vi "MVC OOP Advanced with Commands.vi"() -> ()   [LabVIEW 2011]
doc: "This VI is a basic function generator utilising a class to encapsulate the frequency, type and resulatnt waveform. It also utilises the command pattern design pattern to control the program flow."
uses:
  Controls/Waveform Type.ctl
  Advanced Waveform Class/Advanced Waveform.lvclass
  Message Class/Message.lvclass
  Message Class/Stop Message/Stop Message.lvclass
  Message Class/Set Frequency Message/Set Frequency Message.lvclass
  Message Class/Waveform Type Message/Waveform Type Message.lvclass
  Message Class/Generate Signal Message/Generate Signal Message.lvclass
  Message Class/FFT Signal Message/FFT Signal Message.lvclass
panel:
  in  "Waveform Type":T1
  in  "FFT Signal":bool
  in  "Gen Signal":bool
  in  "Frequency":dbl(knob) scale=0.0..11.0
  out "Waveform Graph":waveform(dbl)(graph)
  in  "stop":bool
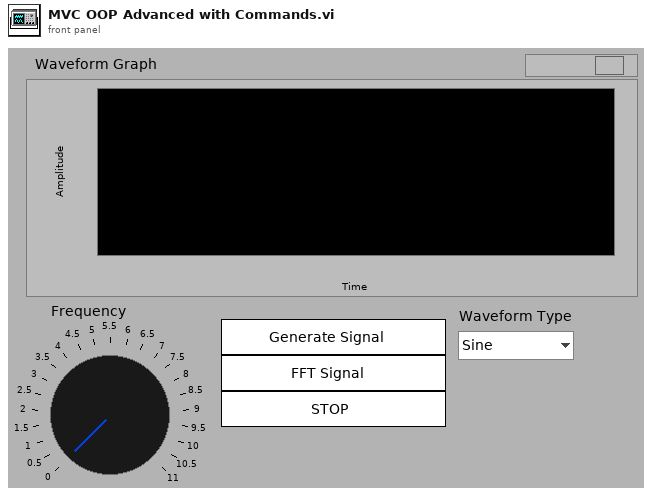
[diagram p1: front panel]
types:
  T1 = typedef "Waveform Type.ctl" = enum16{"Sine", "Square", "Triangle"}
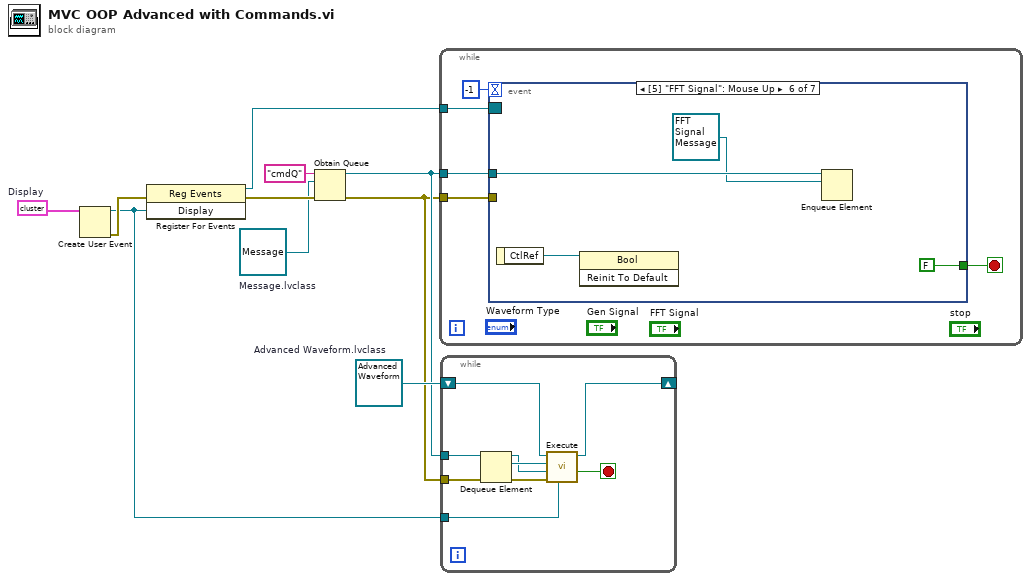
[diagram p0: block diagram]
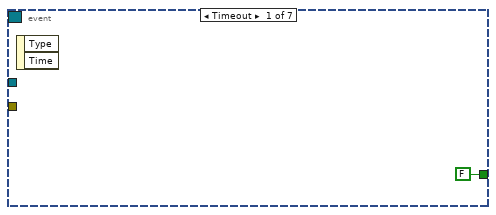
[diagram p2: hidden frame]
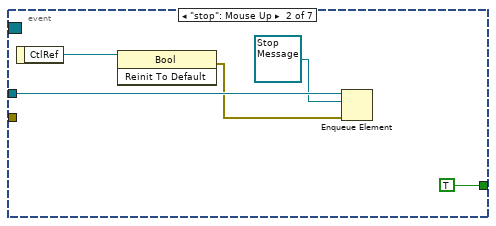
[diagram p3: hidden frame]
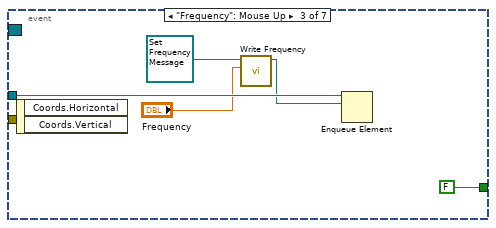
[diagram p4: hidden frame]
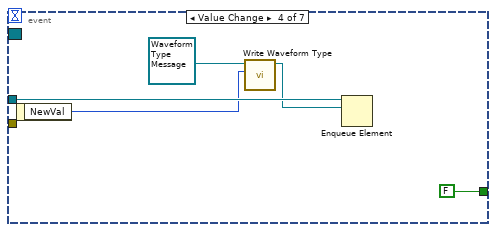
[diagram p5: hidden frame]
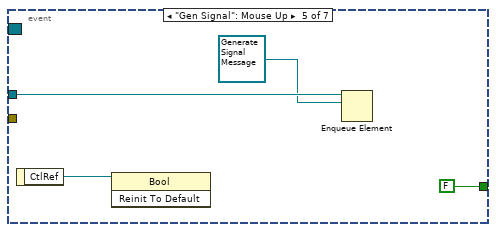
[diagram p6: hidden frame]
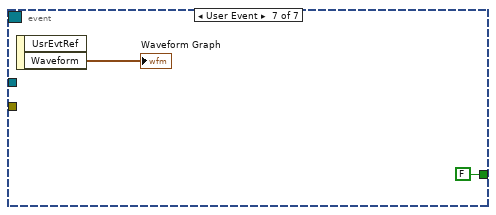
[diagram p7: hidden frame]
diagram:
  w3 = refnum<class "Message.lvclass"> refnum  # Message.lvclass
  w4 = refnum<class "Advanced Waveform.lvclass"> refnum  # Advanced Waveform.lvclass
  w8 = cluster{"Waveform":waveform(dbl)} {"Waveform"={"t0"=timestamp(0 s since 1904-01-01), "dt"=1.0, "Y"=[]}}  # Display
  n1 = Create User Event(user event datatype=w8) -> (user event=w5:refnum<user-event>, error out=w7:errorcluster)  [unwired: 1 in]
  n2 = register-events(error in=w7, w5) -> (reference out=w6:refnum<event-registration>, error out=w9:errorcluster)  [unwired: 1 in]
  n3 = Obtain Queue(name (unnamed)="cmdQ", element data type=w3, error in (no error)=w9) -> (queue out=w2:refnum<queue>, error out=w1:errorcluster)  [unwired: 2 in, 1 out]
  n4 = while {
    tunnel: w2 -> [w14]
    tunnel: w6 -> [w12]
    tunnel: w1 -> [w11]
    stop <- w13 stop-if-true
    n5 = event shown="[5] \"FFT Signal\": Mouse Up" {
      selector: w12 -> [_ _ _ _ _ _ _]
      dyn-events: _ -> [_ _ _ _ _ _ _]
      timeout: -1 -> [_ _ _ _ _ _ _]
      tunnel: w14 -> [_ w20 w26 w31 w35 w39 _]
      tunnel: [FALSE TRUE FALSE FALSE FALSE FALSE FALSE] -> w13
      tunnel: w11 -> [_ _ _ _ _ _ _]
      event Timeout {
        n6 = event-data() -> ()  [unwired: 1 in, 2 out]
      }
      event "stop": Mouse Up {
        n7 = event-data() -> ("CtlRef"=w21:refnum<vi>)  [unwired: 1 in]
        n8 = invoke class="Bool" method="Reinit To Default"(reference=w21) -> (error out=w19:errorcluster)  [unwired: 2 in, 2 out]
        n9 = Enqueue Element(queue=w20, element=refnum<class "Stop Message.lvclass"> refnum ("Stop Message.lvclass"), error in (no error)=w19) -> ()  [unwired: 1 in, 3 out]
      }
      event "Frequency": Mouse Up {
        n10 = event-data() -> ()  [unwired: 1 in, 2 out]
        n11 = call-dynamic "Write Frequency.vi"("Frequency"="Frequency", "Set Frequency Message in"=refnum<class "Set Frequency Message.lvclass"> refnum ("Set Frequency Message.lvclass")) -> ("Set Frequency Message out"=w22:refnum<class "Set Frequency Message.lvclass">)  [unwired: 8 in, 1 out]
        n12 = Enqueue Element(queue=w26, element=w22) -> ()  [unwired: 2 in, 3 out]
      }
      event Value Change {
        n13 = event-data() -> ("NewVal"=w28:T1)  [unwired: 1 in]
        n14 = call-dynamic "Write Waveform Type.vi"("Waveform Type"=w28, "Waveform Type Message in"=refnum<class "Waveform Type Message.lvclass"> refnum ("Waveform Type Message.lvclass")) -> ("Waveform Type Message out"=w27:refnum<class "Waveform Type Message.lvclass">)  [unwired: 8 in, 1 out]
        n15 = Enqueue Element(queue=w31, element=w27) -> ()  [unwired: 2 in, 3 out]
      }
      event "Gen Signal": Mouse Up {
        n16 = event-data() -> ("CtlRef"=w33:refnum<vi>)  [unwired: 1 in]
        n17 = invoke class="Bool" method="Reinit To Default"(reference=w33) -> ()  [unwired: 2 in, 3 out]
        n18 = Enqueue Element(queue=w35, element=refnum<class "Generate Signal Message.lvclass"> refnum ("Generate Signal Message.lvclass")) -> ()  [unwired: 2 in, 3 out]
      }
      event "FFT Signal": Mouse Up {
        n19 = event-data() -> ("CtlRef"=w37:refnum<vi>)  [unwired: 1 in]
        n20 = invoke class="Bool" method="Reinit To Default"(reference=w37) -> ()  [unwired: 2 in, 3 out]
        n21 = Enqueue Element(queue=w39, element=refnum<class "FFT Signal Message.lvclass"> refnum ("FFT Signal Message.lvclass")) -> ()  [unwired: 2 in, 3 out]
      }
      event User Event {
        n22 = event-data() -> ("Waveform"=→"Waveform Graph":waveform(dbl))  [unwired: 1 in, 1 out]
      }
    }
  }
  n23 = while {
    tunnel: w1 -> [w49]
    tunnel: w2 -> [w50]
    tunnel: w5 -> [w44]
    shift-right: [w42] -> _
    shift-left: w4 -> [w47]
    stop <- w43 stop-if-true
    n24 = Dequeue Element(queue=w50, error in (no error)=w49) -> (queue out=w45:refnum<queue>, element=w48:refnum<class "Message.lvclass">, error out=w46:errorcluster)  [unwired: 1 in, 1 out]
    n25 = call-dynamic "Execute.vi"("user event in"=w44, "Advanced Waveform In"=w47, "Message in"=w48, "Command Queue"=w45, "error in (no error)"=w46) -> ("Advanced Waveform Out"=w42:refnum<class "Advanced Waveform.lvclass">, "Stop"=w43:bool)  [unwired: 3 in, 2 out]
  }
